vi "setRampRate.vi"(0 "Interface in":T1, 7 "rampRate":sgl, 11 "error in (no error)":errorcluster) -> (4 "Interface out":T1, 15 "error out":errorcluster)   [LabVIEW 2017, in "BuckBoostInterface.lvlib"]
uses:
  BuckBoostInterface.lvlib
  Interface.ctl
  <instrlib>/_niInstr/Instruction Framework/v1/Host/Instruction Target/niInstr Instruction Target v1 Host.lvclass
  <instrlib>/_niInstr/Instruction Framework/v1/Host/Instruction Framework Context/niInstr Instruction Framework Context v1 Host.lvclass
  <vilib>/NI/JSON Support for LabVIEW/JSON Data Classes/JSON Numeric/JSON Numeric.lvclass
  C:/Program Files (x86)/National Instruments/LabVIEW 2017/vi.lib/NI/JSON Support for LabVIEW/JSON Data Classes/JSON Datatype/JSON Null.lvclass
  <vilib>/NI/JSON Support for LabVIEW/JSON Data Classes/JSON Numeric/New JSON Numeric.vi
  <vilib>/NI/JSON Support for LabVIEW/JSON Data Classes/JSON Object/New JSON Object (Empty).vi
  <vilib>/NI/JSON Support for LabVIEW/JSON Data Classes/JSON Object/Insert Key Value Pair (Single).vi
  <vilib>/NI/JSON Support for LabVIEW/JSON Data Classes/JSON Helper/Parsing/Parse Value.vi
  <vilib>/NI/JSON Support for LabVIEW/JSON Data Classes/JSON Helper/To More Specific Type (Object).vi
  <vilib>/NI/JSON Support for LabVIEW/JSON Data Classes/JSON Datatype/JSON Null.lvclass
  <vilib>/NI/JSON Support for LabVIEW/JSON Data Classes/JSON Object/JSON Object.lvclass
  <vilib>/NI/JSON Support for LabVIEW/JSON Data Classes/JSON Helper/JSON Helper.lvclass
  C:/Program Files (x86)/National Instruments/LabVIEW 2017/vi.lib/NI/JSON Support for LabVIEW/JSON Data Classes/JSON Basic Type/JSON Literal.lvclass
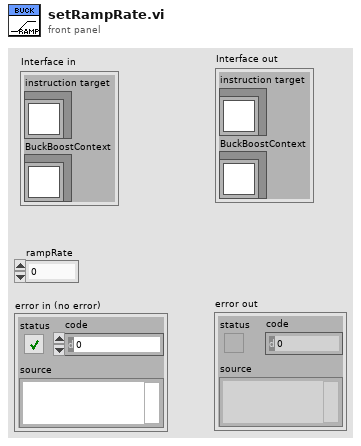
[diagram p1: front panel]
types:
  T1 = typedef "BuckBoostInterface.lvlib/Interface.ctl" = cluster{"instruction target":refnum<class "niInstr Instruction Target v1 Host.lvclass">, "BuckBoostContext":refnum<class "niInstr Instruction Framework Context v1 Host.lvclass">}
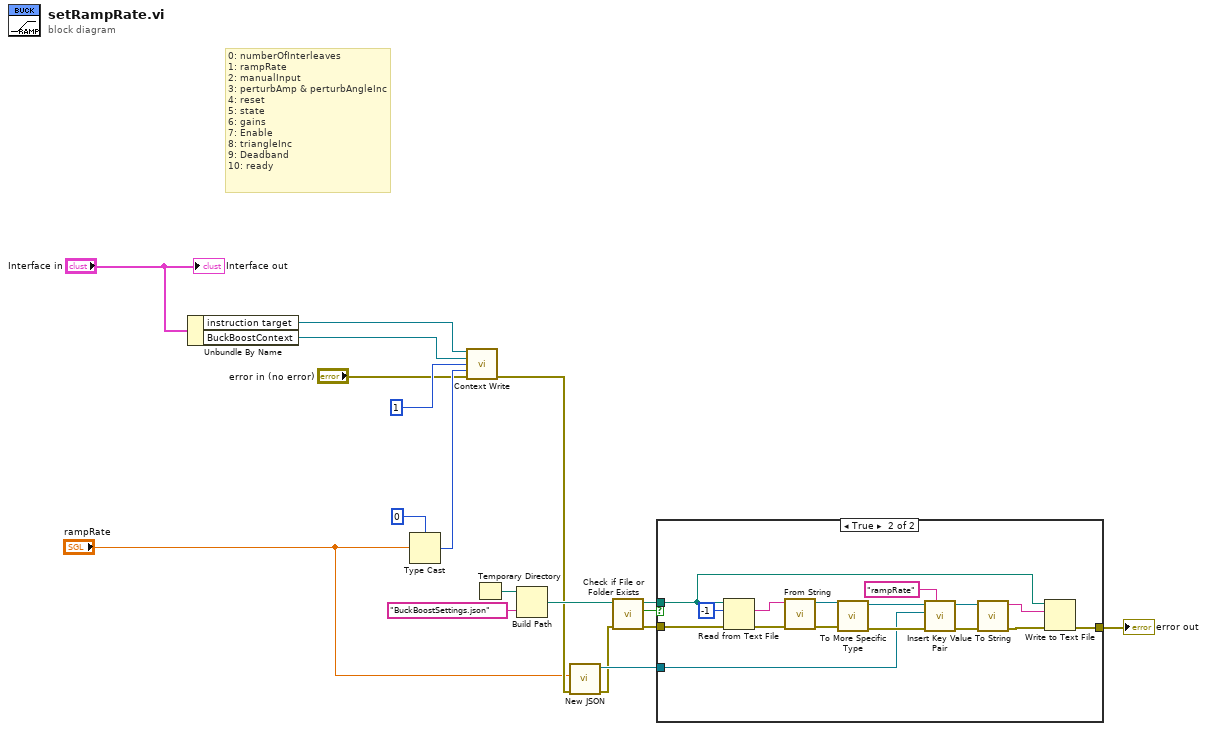
[diagram p0: block diagram]
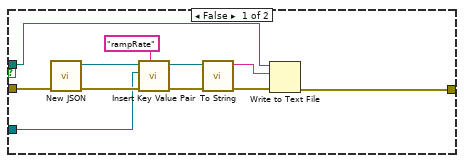
[diagram p2: hidden frame]
diagram:
  # "0: numberOfInterleaves\n1: rampRate\n2: manualInput\n3: perturbAmp & perturbAngleInc\n4: reset\n5: state\n6: gains\n7: Enable\n8: triangleInc\n9: Deadband\n10: ready"
  n1 = Unbundle By Name("Interface in") -> ("instruction target"=w13:refnum<class "niInstr Instruction Target v1 Host.lvclass">, "BuckBoostContext"=w12:refnum<class "niInstr Instruction Framework Context v1 Host.lvclass">)
  n2 = Type Cast(type=u32 0, x="rampRate") -> (*(type *) &x=w18:u32)
  n3 = call <instrlib>:"Context Write.vi"("instruction target in"=w13, "context in"=w12, "address"=u64 1, "data"=w18, "error in"="error in (no error)") -> ("error out"=w3:errorcluster)  [unwired: 8 in, 2 out]
  n4 = Temporary Directory() -> (w11:path)
  n5 = Build Path(base path=w11, name or relative path="BuckBoostSettings.json") -> (appended path=w9:path)
  n6 = call-poly <vilib>:"New JSON.vi"("error in (no error)"=w3, "value"="rampRate") -> ("error out"=w4:errorcluster, "JSON String out"=w6:refnum<class "JSON Numeric.lvclass">)  [unwired: 8 in]
  n7 = call <vilib>:"Check if File or Folder Exists.vi"("error in (no error)"=w4, "path"=w9) -> ("error out"=w5:errorcluster, "file or folder exists?"=w7:bool, "dup path"=w8:path)  [unwired: 7 in]
  n8 = case shown="True" w7 {
    tunnel: w8 -> [w24 w36]
    tunnel: w6 -> [w26 w38]
    tunnel: w5 -> [w29 w37]
    tunnel: [w23 w31] -> w1
    frame False {
      n9 = call-poly <vilib>:"New JSON.vi"("error in (no error)"=w29) -> ("error out"=w27:errorcluster, "JSON Object out"=w28:refnum<class "JSON Object.lvclass">)  [unwired: 9 in]
      n10 = call-poly <vilib>:"Insert Key Value Pair.vi"("key"="rampRate", "error in (no error)"=w27, "value"=w26, "JSON Object in"=w28) -> ("error out"=w22:errorcluster, "JSON Object out"=w19:refnum<class "JSON Object.lvclass">)  [unwired: 5 in, 1 out]
      n11 = call-dynamic "To String.vi"("error in (no error)"=w22, "JSON Object in"=w19) -> ("error out"=w21:errorcluster, "String"=w20:string)  [unwired: 8 in]
      n12 = Write to Text File(file (use dialog)=w24, text=w20, error in=w21) -> (error out=w23:errorcluster)  [unwired: 1 in, 2 out]
    }
    frame True {
      n13 = Read from Text File(file (use dialog)=w36, count=-1, error in=w37) -> (text=w45:string, error out=w40:errorcluster)  [unwired: 1 in, 2 out]
      n14 = call <vilib>:"From String.vi"("error in (no error)"=w40, "JSON String"=w45) -> ("error out"=w44:errorcluster, "JSON out"=w43:refnum<class "JSON Null.lvclass">)  [unwired: 8 in]
      n15 = call-poly <vilib>:"To More Specific Type.vi"("error in (no error)"=w44, "JSON Datatype in"=w43) -> ("error out"=w41:errorcluster, "JSON Datatype out"=w42:refnum<class "JSON Object.lvclass">)  [unwired: 8 in]
      n16 = call-poly <vilib>:"Insert Key Value Pair.vi"("key"="rampRate", "error in (no error)"=w41, "value"=w38, "JSON Object in"=w42) -> ("error out"=w33:errorcluster, "JSON Object out"=w35:refnum<class "JSON Object.lvclass">)  [unwired: 5 in, 1 out]
      n17 = call-dynamic "To String.vi"("error in (no error)"=w33, "JSON Object in"=w35) -> ("error out"=w32:errorcluster, "String"=w34:string)  [unwired: 8 in]
      n18 = Write to Text File(file (use dialog)=w36, text=w34, error in=w32) -> (error out=w31:errorcluster)  [unwired: 1 in, 2 out]
    }
  }
  "error out" <- w1
  "Interface out" <- "Interface in"
